vi "Calibration File Locate.vi"(11 "Base Path":path) -> (0 "Singing Helmet Calibration":path, 1 "SPL Calibration":path, 2 "Flow Calibration":path, 3 "Pressure Calibration":path)   [LabVIEW 2020, in "CollectionSupport.lvlib"]
uses:
  CollectionSupport.lvlib
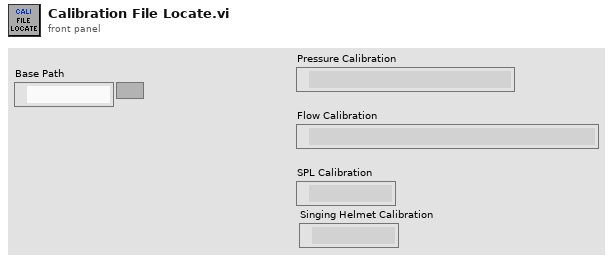
[diagram p1: front panel]
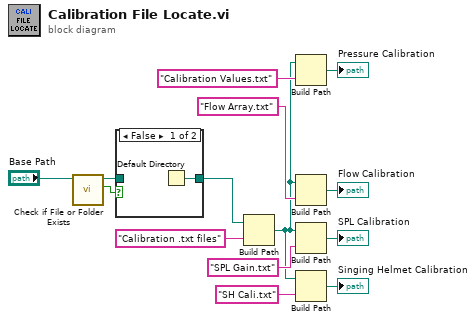
[diagram p0: block diagram]
diagram:
  n1 = call <vilib>:"Check if File or Folder Exists.vi"("path"="Base Path") -> ("file or folder exists?"=w6:bool, "dup path"=w5:path)  [unwired: 8 in, 1 out]
  n2 = case shown="False" w6 {
    tunnel: w5 -> [_ w16]
    tunnel: [w15 w16] -> w4
    frame False {
      n3 = Default Directory() -> (w15:path)
    }
    frame True {
    }
  }
  n4 = Build Path(base path=w4, name or relative path="Calibration .txt files") -> (appended path=w3:path)
  n5 = Build Path(base path=w3, name or relative path="Calibration Values.txt") -> (appended path=→"Pressure Calibration":path)
  n6 = Build Path(base path=w3, name or relative path="Flow Array.txt") -> (appended path=→"Flow Calibration":path)
  n7 = Build Path(base path=w3, name or relative path="SPL Gain.txt") -> (appended path=→"SPL Calibration":path)
  n8 = Build Path(base path=w3, name or relative path="SH Cali.txt") -> (appended path=→"Singing Helmet Calibration":path)
